vi "GetProcessInstanceRef.vi"(8 "error in (no error)":errorcluster, 10 "Process Name":string, 11 "SMO":refnum<class "SMO.lvclass">) -> (0 "error out":errorcluster, 2 "Process VI Refnum":refnum<vi>, 3 "SMO out":refnum<class "SMO.lvclass">)   [LabVIEW 2013, in "SMO.lvclass"]
doc: "This method will lookup (and return) the instance reference of <b>Process Name</b>.\n\n---------------------------------------------------------------\nJKI State Machine Objects™\nhttp://jki.net/state-machine-objects/\nCopyright (C) 2005-2015, JKI <info@jki.net>\nALL RIGHTS RESERVED"
uses:
  SMO.lvclass
  SMO.lvclass/SMO.ctl
panel:
  # "For instructions on how to use the JKI State Machine Objects, examples and video tutorials, visit:\nhttp://jki.net/state-machine-objects/\n\nJKI State Machine Objects™\nhttp://jki.net/state-machine-objects/\nCopyright (C) 2005-2015, JKI <info@jki.net>\nALL RIGHTS RESERVED"
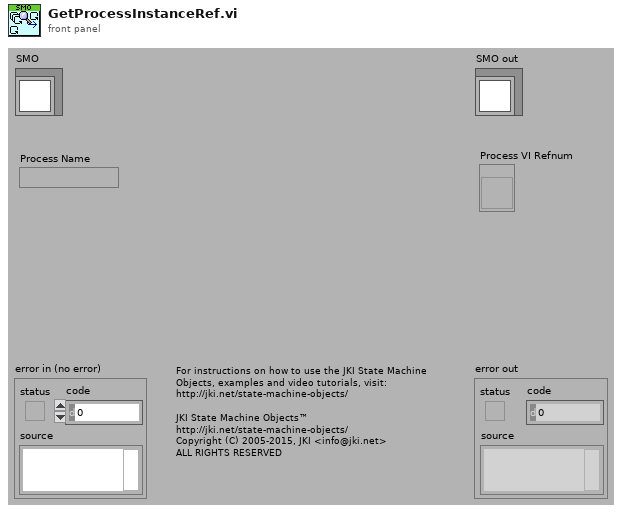
[diagram p1: front panel]
types:
  T1 = typedef "SMO.lvclass/PrivateData--Ref.ctl" = refnum<data-value>
  T2 = typedef "SMO.lvclass/PrivateData--Cluster.ctl" = cluster{"Parent Call":T3, "Registered Processes":T4[], "Sync Notifier":refnum<notifier>, "Process Error Notifier":refnum<notifier>, "Protected Events":T5, "Public Events":T6, "SMO State":T7, "[Attributes]":variant, "Launcher Close":refnum<notifier>, "Caller Watchdog":refnum<queue>, "Accessibility":T8, "NbStaticDependencies":u32}
  T3 = typedef "SMO.lvclass/Parent Call--Enum.ctl" = enum16{"Allows parent to run", "Does not request parent to run"}
  T4 = typedef "SMO.lvclass/RegisteredProcessData--Cluster.ctl" = cluster{"Name":string, "Static VI Ref":refnum<vi>, "Running":bool, "NotifierRef":u32}
  T5 = typedef "SMO.lvclass/Protected Events.ctl" = cluster{"StopProcesses":refnum<user-event>, "AbortProcesses":refnum<user-event>, "Config Changed":refnum<user-event>, "Dependency":refnum<user-event>}
  T6 = typedef "SMO.lvclass/Public Events.ctl" = cluster{"Error":refnum<user-event>, "State":refnum<user-event>, "Reserve State":refnum<user-event>}
  T7 = typedef "SMO.lvclass/SMOState --Enum.ctl" = enum16{"unknown", "Created", "Started", "Stopped"}
  T8 = typedef "SMO.lvclass/Accessibility--Cluster.ctl" = cluster{"Lock Key":string, "Reserve State":T9}
  T9 = typedef "SMO.lvclass/Reserve State--Enum.ctl" = enum16{"Unreserved", "Reserved", "Self-locked"}
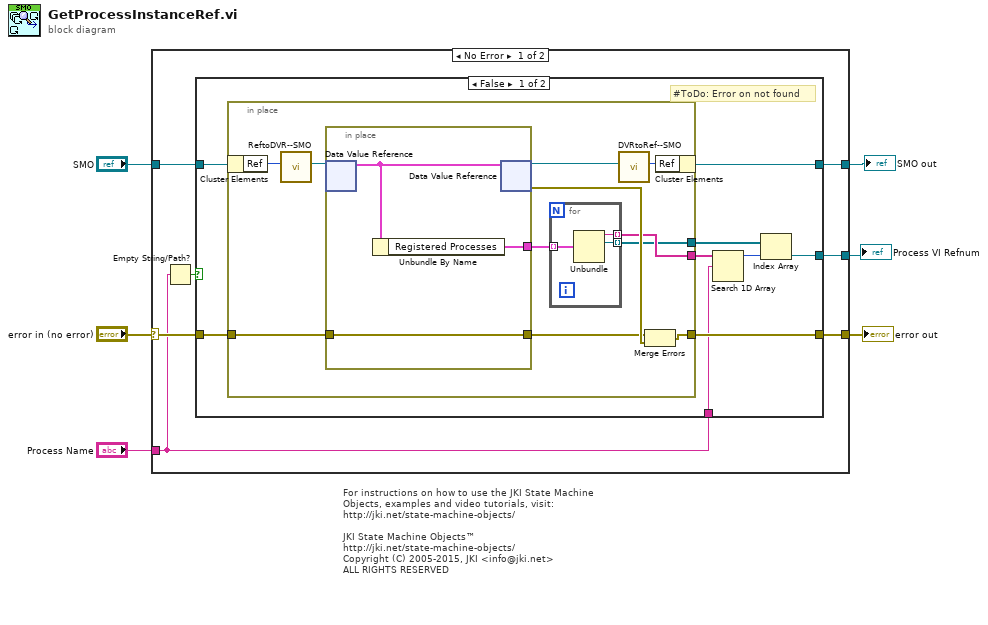
[diagram p0: block diagram]
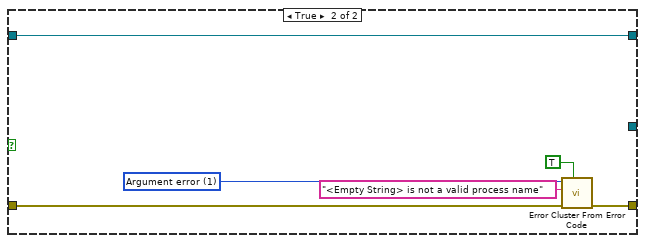
[diagram p2: hidden frame]
diagram:
  # "For instructions on how to use the JKI State Machine Objects, examples and video tutorials, visit:\nhttp://jki.net/state-machine-objects/\n\nJKI State Machine Objects™\nhttp://jki.net/state-machine-objects/\nCopyright (C) 2005-2015, JKI <info@jki.net>\nALL RIGHTS RESERVED"
  n1 = case shown="No Error" "error in (no error)" {
    selector: "error in (no error)" -> [w12 w47]
    tunnel: [w11 w47] -> w1
    tunnel: [w10 w46] -> w2
    tunnel: "SMO" -> [w13 w46]
    tunnel: [w9 _] -> w3
    tunnel: "Process Name" -> [w7 _]
    frame No Error {
      n2 = Empty String/Path?(string/path=w7) -> (empty?=w8:bool)
      n3 = case shown="False" w8 {
        tunnel: w13 -> [w22 w45]
        tunnel: w12 -> [w21 w43]
        tunnel: [w20 w42] -> w11
        tunnel: [w19 w45] -> w10
        tunnel: [w15 _] -> w9
        tunnel: w7 -> [w18 _]
        frame False {
          # "#ToDo: Error on not found"
          n4 = in-place {
            in-place-border: w21 -> [w33]
            in-place-border: [w30] -> w20
            in-place-border: [w27] -> w16
            in-place-border: [w28] -> w14
            n5 = in-place-cluster #1(w22) -> ("Ref"=w24:u32)
            n6 = call "ReftoDVR--SMO.vi"("Ref"=w24) -> ("Ref"=w23:T1)  [unwired: 10 in]
            n7 = in-place {
              in-place-border: w33 -> [w38]
              in-place-border: [w38] -> w31
              in-place-border: [w37] -> w29
              n8 = in-place-dvr #2(w23) -> (w39:T2)  [unwired: 1 out]
              n9 = Unbundle By Name(w39) -> ("Registered Processes"=w37:T4[])
              n10 = in-place-dvr #2(w39) -> (w26:T1, w32:errorcluster)
            }
            n11 = for {
              tunnel: w29 -> [w36] mode=indexing
              tunnel: [w35] -> w28 mode=indexing
              tunnel: [w34] -> w27 mode=indexing
              n12 = Unbundle(w36) -> ("Name"=w35:string, "Static VI Ref"=w34:refnum<vi>)  [unwired: 2 out]
            }
            n13 = call "DVRtoRef--SMO.vi"("Ref"=w26) -> ("Ref"=w25:u32)  [unwired: 10 in]
            n14 = Merge Errors(w31, w32) -> (w30:errorcluster)
            n15 = in-place-cluster #1("Ref"=w25) -> (w19:refnum<class "SMO.lvclass">)
          }
          n16 = Search 1D Array(1D array=w14, element=w18) -> (index of element=w17:i32)  [unwired: 1 in]
          n17 = Index Array(array=w16, index=w17) -> (element=w15:refnum<vi>)
        }
        frame True {
          w44 = 1 items=["No error", "Argument error", "Memory is full", "Out of zone", "End of file", "File already open", "Generic file I/O error", "File not found", "File permission error", "Disk is full", "Duplicate path", "Too many files open", "System feature not enabled", "Resource file not found", "Cannot add resource", "Resource not found", "Image not found", "Image memory error", "Pen does not exist", "Config type invalid", "Config token not found", "Config parse error", "Config memory error", "Bad external code format", "Bad external code offset", "External code not present", "Null window", "Destroy window error", "Null menu", "Print aborted", "Bad print record", "Print driver error", "Windows error during printing", "Memory error during printing", "Print dialog error", "Generic print error", "Invalid device refnum", "Device not found", "Device parameter error", "Device unit error", "Cannot open device", "Device call aborted", "Generic error", "Cancelled by user", "Object ID too low", "Object ID too high", "Object not in heap", "Unknown heap", "Unknown object (invalid DefProc)", "Unknown object (DefProc not in table)", "Message out of range", "Invalid (null) method", "Unknown message", "Manager call not supported", "Bad address", "Network operation in progress", "Network operation timed out", "Connection is busy", "Network attribute not supported", "Network error", "Address in use", "System out of memory", "Connection aborted", "Connection refused", "Not connected", "Already connected", "Connection closed", "Initialization error (interapplication manager)", "Bad occurrence", "Wait on unbound occurrence handler", "Occurrence queue overflow", "Datalog type conflict", "Unused", "Unrecognized type (interapplication manager)", "Memory corrupt", "Failed to make temporary DLL", "Old CIN version", "Drag socket not found", "Failed to load drop-object", "Failed to register OLE object", "Failed to release OLE object", "Format specifier type mismatch", "Unknown format specifier", "Too few format specifiers", "Too many format specifiers", "Scan failed", "Newer CIN version", "Error converting to variant", "Runtime menu error", "Password tampered", "Variant attribute not found", "Incompatible variant data type", "Event data is not available", "Event Store is not present", "Occurrence is not found", "Event Queue is not created", "Event info is not available", "Refnum passed is NULL", "Error retrieving Class GUID", "Error retrieving CoClass GUID", "Error retrieving TypeLib GUID.", "Bad built application magic bytes.", "Specific driver is different from the specific driver associated with the Logical Name.", "There is no session opened to the class driver.", "Max Error", "MAX - Error with config objects", "MAX - Error loading configuration", "MAX - Group not supported"]
          n18 = call <vilib>:"Error Cluster From Error Code.vi"("show call chain? (False)"=TRUE, "error in (no error)"=w43, "error message (\"\")"="<Empty String> is not a valid process name" ("error message (\"\")"), "error code (0)"=w44) -> ("error out"=w42:errorcluster)  [unwired: 5 in]
        }
      }
    }
    frame Error {
    }
  }
  "error out" <- w1
  "SMO out" <- w2
  "Process VI Refnum" <- w3
